vi "Draw.vi"(8 "Error In":errorcluster, 10 "PictureIn":picture, 11 "object in":refnum<class "Circle.lvclass">) -> (0 "Error Out":errorcluster, 2 "PictureOut":picture, 3 "object out":refnum<class "Circle.lvclass">)   [LabVIEW 2020, in "Circle.lvclass"]
uses:
  Circle.lvclass
  Circle.lvclass/Circle.ctl
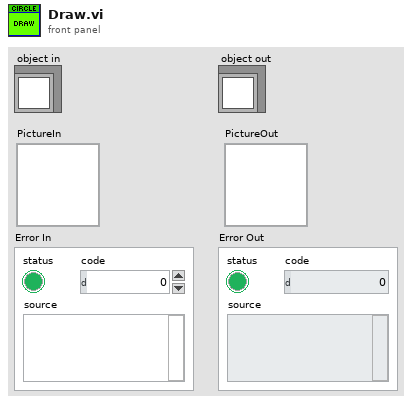
[diagram p1: front panel]
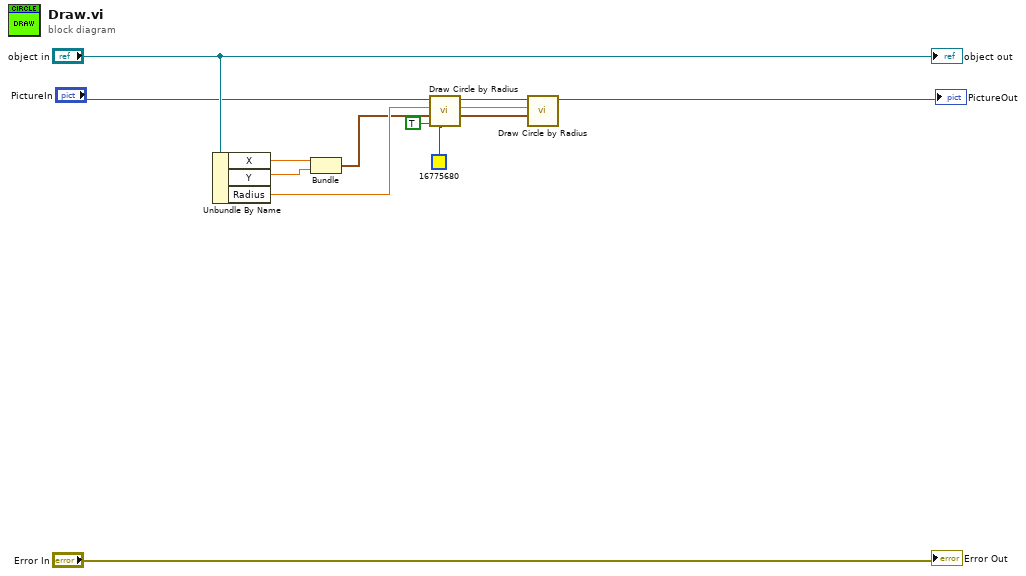
[diagram p0: block diagram]
diagram:
  n1 = Unbundle By Name("object in") -> ("X"=w7:dbl, "Y"=w6:dbl, "Radius"=w3:dbl)
  n2 = Bundle("X"=w7, "Y"=w6) -> (w2:cluster{"X":dbl, "Y":dbl})  [unwired: 1 in]
  n3 = call <vilib>:"Draw Circle by Radius.vi"("color(black)"=u32 16775680, "fill?(F)"=TRUE, "pixel center"=w2, "radius"=w3, "picture"="PictureIn") -> ("new picture"=w4:picture)  [unwired: 6 in]
  n4 = call <vilib>:"Draw Circle by Radius.vi"("pixel center"=w2, "radius"=w3, "picture"=w4) -> ("new picture"=→"PictureOut":picture)  [unwired: 8 in]
  "Error Out" <- "Error In"
  "object out" <- "object in"
